vi "Control_MoveSnakeHead.vi"(1 "InputLeft":bool, 4 "InputRight":bool, 6 "InitialDirection":T3=enum."Right", 8 "InitialPosition":i16, 9 "Reset":bool, 10 "Player":T2) -> (15 "PickUp":T1, 18 "PlayerDied?":bool)   [LabVIEW 2018]
uses:
  TypDefs/Direction_Enum.ctl
  TypDefs/Player_Enum.ctl
  TypDefs/Tile_Enum.ctl
  <vilib>/rvi/DataTransferAndStorage/Container/Common/niFpgaContainerExecOnDevCompGetState.vi
  <vilib>/rvi/Emulation/niFpgaEmulationIsFPGAContextNoSignature.vi
  <vilib>/rvi/DataTransferAndStorage/Container/Common/niFpgaContainerGetUniqueNameForEmu.vi
  <vilib>/rvi/Emulation/niFpgaProcessEmulError.vi
  <vilib>/rvi/Emulation/niFpgaSctlEmulationGetInTimedLoop.vi
  <vilib>/rvi/errors/nirviReportUnexpectedCaseInternalError (U32).vi
  <vilib>/rvi/Memory/Memory_Emulation/niFpgaMemoryEmulationCacheClearOnFirstRun.vi
  <vilib>/rvi/Memory/Memory_Emulation/nirvimemoryEmulationManagerCache_MakeExclusive.vi
  <vilib>/rvi/Memory/Memory_Emulation/niFpgaMemoryEmulationValidateCache.vi
  <vilib>/rvi/Memory/Memory_Emulation/nirvimemoryEmulationManagerCache_InsertValue.vi
  <vilib>/Utility/error.llb/Clear Errors.vi
  <vilib>/rvi/Memory/Memory_Emulation/nirvimemoryEmulationManagerCache_ReleaseExclusive.vi
  <vilib>/rvi/Memory/Memory_Emulation/nirvimemoryEmulationManagerCache_GetValue.vi
  <vilib>/rvi/Memory/Memory_Emulation/nirvimemoryEmulationManagerCache_SetValue.vi
  <vilib>/rvi/Emulation/niFpgaSctlEmulationResourceMgr.vi
  <vilib>/rvi/DataTransferAndStorage/Container/XNode/niFpgaContainer.xnode
  <vilib>/rvi/Memory/Memory_Emulation/niFpgaMemoryEmulationRefIn.vi
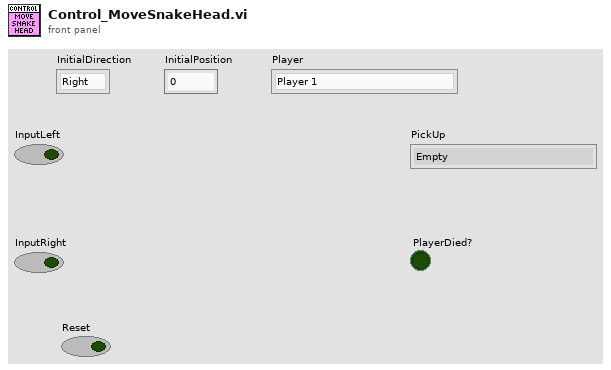
[diagram p1: front panel]
types:
  T1 = typedef "Tile_Enum.ctl" = enum8{"Empty", "Snake1_HeadPointingUp", "Snake1_HeadPointingDown", "Snake1_HeadPointingLeft", "Snake1_HeadPointingRight", "Snake1_DeadPointingUp", "Snake1_DeadPointingDown", "Snake1_DeadPointingLeft", "Snake1_DeadPointingRight", "Snake1_TailPointingUp", "Snake1_TailPointingDown", "Snake1_TailPointingLeft", "Snake1_TailPointingRight", "Snake1_Horizontal", "Snake1_Vertical", "Snake1_UpperLeftCorner", "Snake1_UpperRightCorner", "Snake1_LowerLeftCorner", "Snake1_LowerRightCorner", "Snake2_HeadPointingUp", "Snake2_HeadPointingDown", "Snake2_HeadPointingLeft", "Snake2_HeadPointingRight", "Snake2_DeadPointingUp", "Snake2_DeadPointingDown", "Snake2_DeadPointingLeft", "Snake2_DeadPointingRight", "Snake2_TailPointingUp", "Snake2_TailPointingDown", "Snake2_TailPointingLeft", "Snake2_TailPointingRight", "Snake2_Horizontal", "Snake2_Vertical", "Snake2_UpperLeftCorner", "Snake2_UpperRightCorner", "Snake2_LowerLeftCorner", "Snake2_LowerRightCorner", "Wall_Horizontal", "Wall_Vertical", "Wall_UpperLeftCorner", "Wall_UpperRightCorner", "Wall_LowerLeftCorner", "Wall_LowerRightCorner", "Pickup_SpeedUp", "Pickup_Stop", "Pickup_Item1", "Pickup_Item2", "Pickup_Item3", "Pickup_Item4", "Pickup_Item5", "Pickup_Item6"}
  T2 = typedef "Player_Enum.ctl" = enum16{"Player 1", "Player 2"}
  T3 = typedef "Direction_Enum.ctl" = enum8{"Left", "Right", "Up", "Down"}
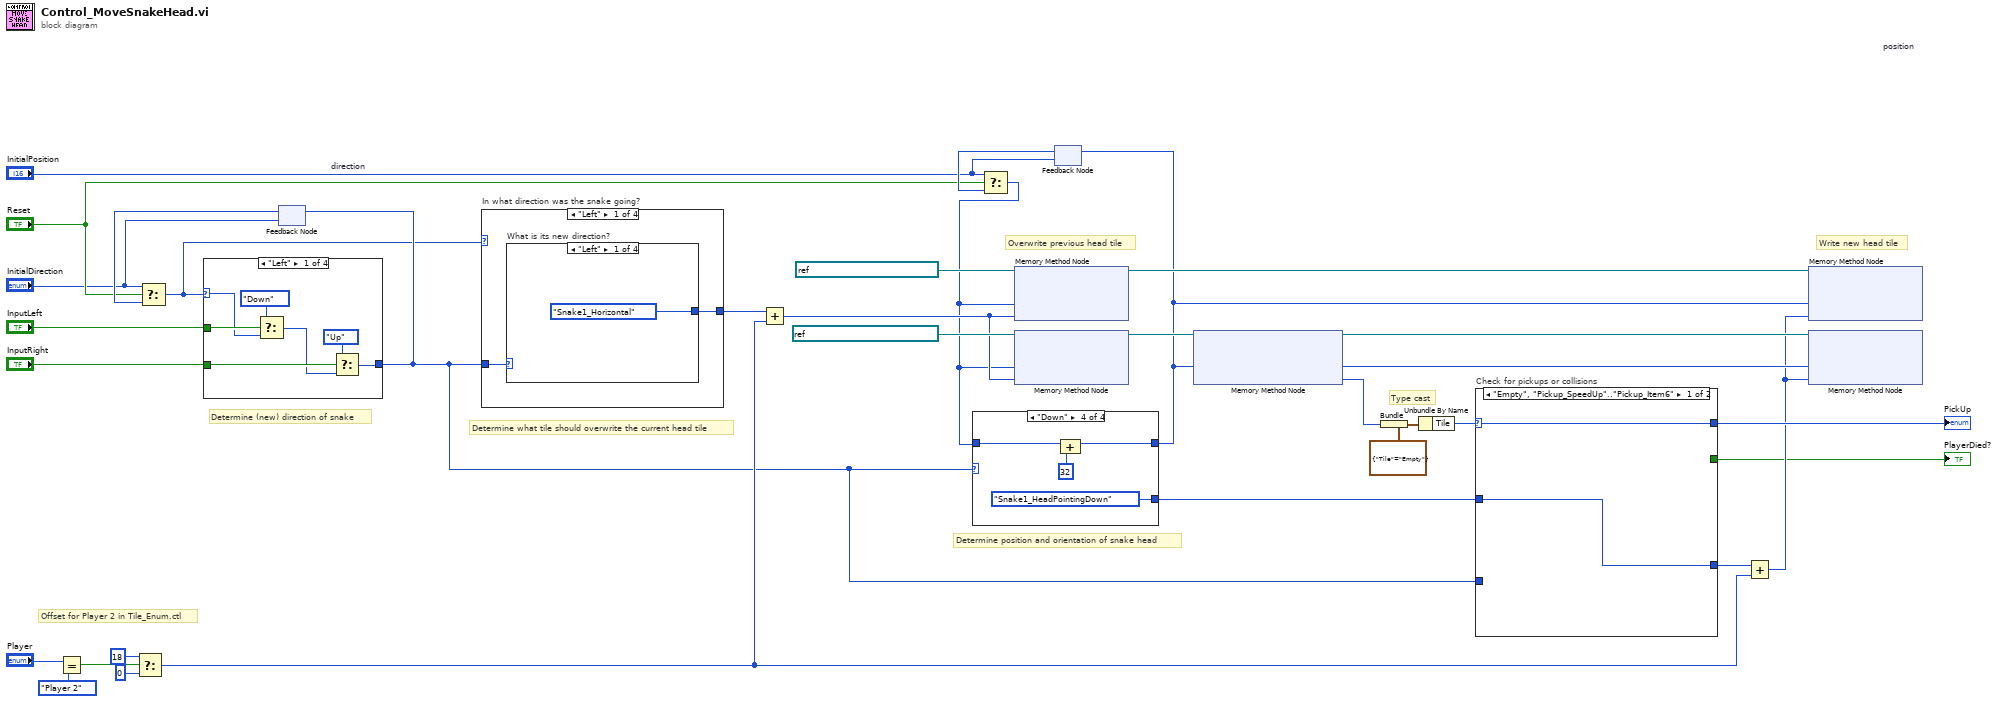
[diagram p0: block diagram]
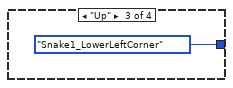
[diagram p3: hidden frame]
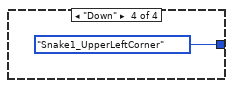
[diagram p4: hidden frame]
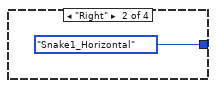
[diagram p6: hidden frame]
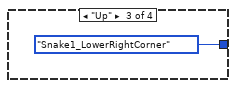
[diagram p7: hidden frame]
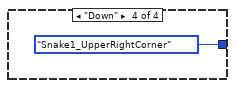
[diagram p8: hidden frame]
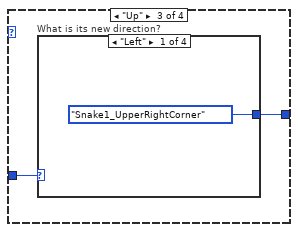
[diagram p9: hidden frame]
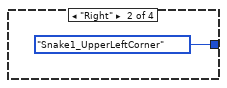
[diagram p10: hidden frame]
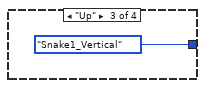
[diagram p11: hidden frame]
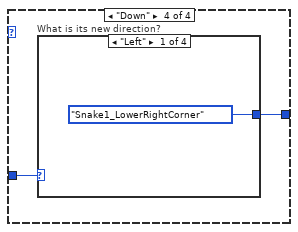
[diagram p13: hidden frame]
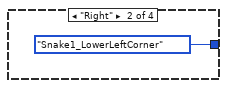
[diagram p14: hidden frame]
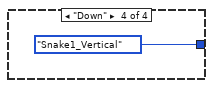
[diagram p16: hidden frame]
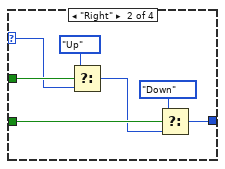
[diagram p17: hidden frame]
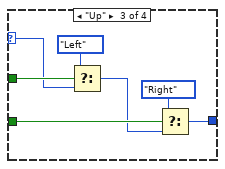
[diagram p18: hidden frame]
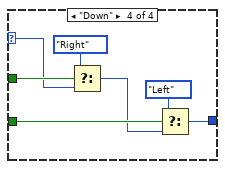
[diagram p19: hidden frame]
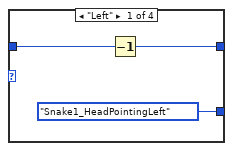
[diagram p20: hidden frame]
diagram:
  # "Offset for Player 2 in Tile_Enum.ctl"
  # "Write new head tile"
  # "Overwrite previous head tile"
  # "Type cast"
  # "Determine position and orientation of snake head"
  # "Determine what tile should overwrite the current head tile"
  # "Determine (new) direction of snake"
  n1 = Equal?(x="Player", y=Player_Enum."Player 2") -> (x = y?=w24:bool)
  n2 = Select(t=u8 18, s=w24, f=u8 0) -> (s? t:f=w11:u8)
  n3 = feedback #1 "direction"("InitialDirection") -> (w7:T3)
  n4 = Select(t="InitialDirection", s="Reset", f=w7) -> (s? t:f=w1:T3)
  n5 = case shown="\"Left\"" w1 {
    selector: w1 -> [w39 w46 w53 w60]
    tunnel: "InputLeft" -> [w40 w47 w54 w61]
    tunnel: "InputRight" -> [w38 w45 w52 w59]
    tunnel: [w34 w41 w48 w55] -> w9
    frame "Left" {
      n6 = Select(t=Direction_Enum."Down", s=w40, f=w39) -> (s? t:f=w37:T3)
      n7 = Select(t=Direction_Enum."Up", s=w38, f=w37) -> (s? t:f=w34:T3)
    }
    frame "Right" {
      n8 = Select(t=Direction_Enum."Up", s=w47, f=w46) -> (s? t:f=w44:T3)
      n9 = Select(t=Direction_Enum."Down", s=w45, f=w44) -> (s? t:f=w41:T3)
    }
    frame "Up" {
      n10 = Select(t=Direction_Enum."Left", s=w54, f=w53) -> (s? t:f=w51:T3)
      n11 = Select(t=Direction_Enum."Right", s=w52, f=w51) -> (s? t:f=w48:T3)
    }
    frame "Down" {
      n12 = Select(t=Direction_Enum."Right", s=w61, f=w60) -> (s? t:f=w58:T3)
      n13 = Select(t=Direction_Enum."Left", s=w59, f=w58) -> (s? t:f=w55:T3)
    }
  }
  n14 = feedback-in #1(w9) -> ()
  n15 = case "In what direction was the snake going?" shown="\"Left\"" w1 {
    tunnel: w9 -> [w63 w68 w73 w78]
    tunnel: [w62 w67 w72 w77] -> w28
    frame "Left" {
      n16 = case "What is its new direction?" shown="\"Left\"" w63 {
        tunnel: [Tile_Enum."Snake1_Horizontal" ("Tile") _ Tile_Enum."Snake1_LowerLeftCorner" ("Tile") Tile_Enum."Snake1_UpperLeftCorner" ("Tile")] -> w62
        frame "Left" {
        }
        frame "Right" {
        }
        frame "Up" {
        }
        frame "Down" {
        }
      }
    }
    frame "Right" {
      n17 = case "What is its new direction?" shown="\"Left\"" w68 {
        tunnel: [_ Tile_Enum."Snake1_Horizontal" ("Tile") Tile_Enum."Snake1_LowerRightCorner" ("Tile") Tile_Enum."Snake1_UpperRightCorner" ("Tile")] -> w67
        frame "Left" {
        }
        frame "Right" {
        }
        frame "Up" {
        }
        frame "Down" {
        }
      }
    }
    frame "Up" {
      n18 = case "What is its new direction?" shown="\"Left\"" w73 {
        tunnel: [Tile_Enum."Snake1_UpperRightCorner" ("Tile") Tile_Enum."Snake1_UpperLeftCorner" ("Tile") Tile_Enum."Snake1_Vertical" ("Tile") _] -> w72
        frame "Left" {
        }
        frame "Right" {
        }
        frame "Up" {
        }
        frame "Down" {
        }
      }
    }
    frame "Down" {
      n19 = case "What is its new direction?" shown="\"Left\"" w78 {
        tunnel: [Tile_Enum."Snake1_LowerRightCorner" ("Tile") Tile_Enum."Snake1_LowerLeftCorner" ("Tile") _ Tile_Enum."Snake1_Vertical" ("Tile")] -> w77
        frame "Left" {
        }
        frame "Right" {
        }
        frame "Up" {
        }
        frame "Down" {
        }
      }
    }
  }
  n20 = Add(x=w28, y=w11) -> (x+y=w27:u8)
  n21 = feedback #2 "position"("InitialPosition") -> (w5:i16)
  n22 = Select(t="InitialPosition", s="Reset", f=w5) -> (s? t:f=w6:i16)
  n23 = case shown="\"Down\"" w9 {
    tunnel: [w84 w87 w90 w94] -> w19
    tunnel: [Tile_Enum."Snake1_HeadPointingLeft" ("Tile") Tile_Enum."Snake1_HeadPointingRight" ("Tile") Tile_Enum."Snake1_HeadPointingUp" ("Tile") Tile_Enum."Snake1_HeadPointingDown" ("Tile")] -> w10
    tunnel: w6 -> [w82 w85 w88 w92]
    frame "Left" {
      n24 = Decrement(x=w82) -> (x-1=w84:i16)
    }
    frame "Right" {
      n25 = Increment(x=w85) -> (x+1=w87:i16)
    }
    frame "Up" {
      n26 = Compound Arithmetic op=ADD(w88, i16 -32 ("y")) -> (w90:i16)
    }
    frame "Down" {
      n27 = Compound Arithmetic op=ADD(w92, i16 32 ("y")) -> (w94:i16)
    }
  }
  n28 = xnode ("Memory Method Node")("Address"=w6, "Data"=w27, "Memory In"=refnum<k21> "BlockMem_FastGameMap") -> ("Memory Out"=w31:refnum<k21>)
  n29 = xnode ("Memory Method Node")("Address"=w6, "Data"=w27, "Memory In"=refnum<k21> "BlockMem_SlowGameMap") -> ("Memory Out"=w21:refnum<k21>)
  n30 = feedback-in #2(w19) -> ()
  n31 = xnode ("Memory Method Node")("Address"=w19, "Memory In"=w21) -> ("Data"=w16:u8, "Memory Out"=w20:refnum<k21>)
  n32 = Bundle(cluster=cluster{"Tile":T1} {"Tile"=enum."Empty"}, "Tile"=w16) -> (w17:cluster{"Tile":T1})
  n33 = Unbundle By Name(w17) -> ("Tile"=w15:T1)
  n34 = case "Check for pickups or collisions" shown="\"Empty\", \"Pickup_SpeedUp\"..\"Pickup_Item6\"" w15 {
    selector: w15 -> [w97 _]
    tunnel: [w97 _] -> w14
    tunnel: [_ TRUE] -> w8
    tunnel: [w96 w99] -> w13
    tunnel: w10 -> [w96 _]
    tunnel: w9 -> [_ w98]
    frame "Empty", "Pickup_SpeedUp".."Pickup_Item6" {
    }
    frame Default {
      n35 = case shown="\"Left\"" w98 {
        tunnel: [Tile_Enum."Snake1_DeadPointingLeft" Tile_Enum."Snake1_DeadPointingRight" Tile_Enum."Snake1_DeadPointingUp" Tile_Enum."Snake1_DeadPointingDown"] -> w99
        frame "Left" {
        }
        frame "Right" {
        }
        frame "Up" {
        }
        frame "Down" {
        }
      }
    }
  }
  "PickUp" <- w14
  "PlayerDied?" <- w8
  n36 = Add(x=w13, y=w11) -> (x+y=w12:u8)
  n37 = xnode ("Memory Method Node")("Address"=w19, "Data"=w12, "Memory In"=w31) -> ()  [unwired: 1 out]
  n38 = xnode ("Memory Method Node")("Address"=w19, "Data"=w12, "Memory In"=w20) -> ()  [unwired: 1 out]
